vi "Start Live Mode.vi"(8 "error in (no error)":errorcluster, 10 "Camera Settings":T1={"Exposure Time (ms)"=100.0, "Binning"=enum."2x2", "Scan Mode"=0, "Frames to Acquire"=1000.0, "Pixel Correction"=FALSE, "Frames to Skip"=0, "File Path"=path "", "Duty cycle"=0.0, "ALEX"=FALSE, "Shutter Enable"=[], "fluidics trigger frame"=0, "Bit Depth"=0, "Image Width (px)"=0, "Image Height (px)"=0, "Horizontal Offset (px)"=0, "Vertical Offset (px)"=0} {"fluidics trigger frame" max=60000 step=1; "Exposure Time (ms)" min=1.0 max=10000.0 step=1.0}, 11 "Photometrics Camera in":refnum<class "Photometrics Camera.lvclass">) -> (0 "error out":errorcluster, 3 "Photometrics Camera out":refnum<class "Photometrics Camera.lvclass">)   [LabVIEW 2022 SP3, in "Photometrics Camera.lvlib" / "Photometrics Camera.lvclass"]
uses:
  Photometrics Camera.lvclass
  Resources/Type Defs/Camera Settings.ctl
  C:/FlashGordon/Development/dll/PVCamNET.dll
  dll/PVCamNET.dll
  Camera/Camera.lvclass
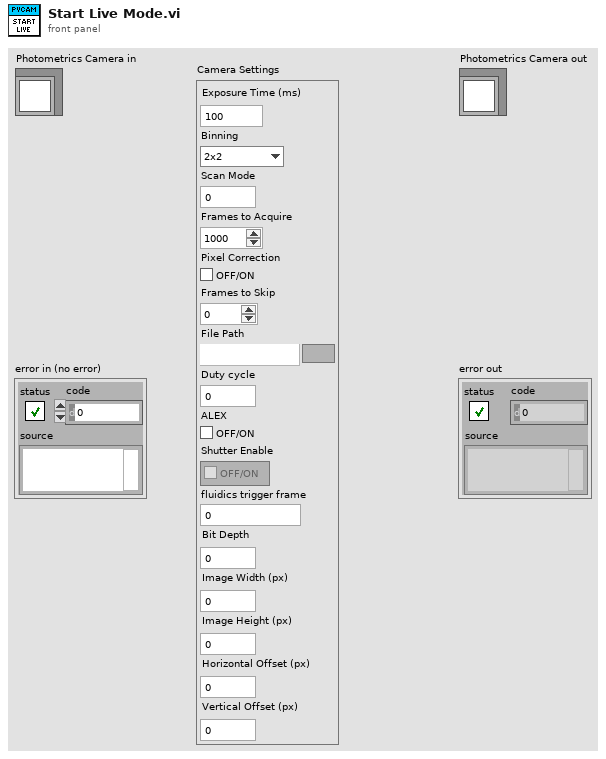
[diagram p1: front panel]
types:
  T1 = typedef "Camera Settings.ctl" = cluster{"Exposure Time (ms)":dbl, "Binning":enum16{"1x1", "2x2", "4x4"}, "Scan Mode":i32, "Frames to Acquire":dbl, "Pixel Correction":bool, "Frames to Skip":u32, "File Path":path, "Duty cycle":dbl, "ALEX":bool, "Shutter Enable":bool[], "fluidics trigger frame":u16, "Bit Depth":u16, "Image Width (px)":u16, "Image Height (px)":u16, "Horizontal Offset (px)":u16, "Vertical Offset (px)":u16}
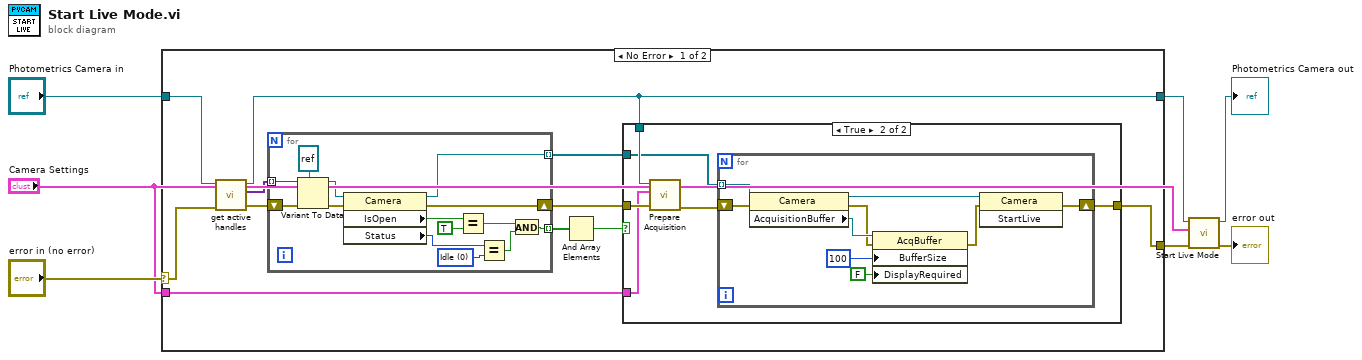
[diagram p0: block diagram]
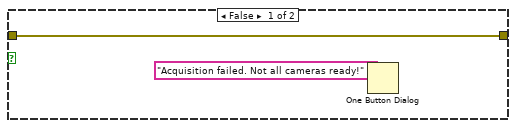
[diagram p2: hidden frame]
diagram:
  n1 = case shown="No Error" "error in (no error)" {
    selector: "error in (no error)" -> [w12 w51]
    tunnel: [w15 w51] -> w3
    tunnel: "Photometrics Camera in" -> [w11 w50]
    tunnel: [w10 w50] -> w2
    tunnel: "Camera Settings" -> [w14 _]
    frame No Error {
      n2 = call-dynamic "get active handles.vi"("error in (no error)"=w12, "Camera in"=w11) -> ("error out"=w13:errorcluster, "Handles"=w9:variant[], "Camera out"=w10:refnum<class "Photometrics Camera.lvclass">)  [unwired: 5 in, 2 out]
      n3 = for {
        tunnel: [w43] -> w17 mode=indexing
        tunnel: w9 -> [w40] mode=indexing
        shift-right: [w42] -> w18
        shift-left: w13 -> [w39]
        tunnel: [w41] -> w8 mode=indexing
        w48 = 0 items=["Idle", "Capturing"] ("Status")
        n4 = Variant To Data(error in=w39, type=refnum<k24> refnum ("reference out"), Variant=w40) -> (data=w37:refnum<k24>, error out=w38:errorcluster)
        n5 = property class="Camera"(reference=w37, error in=w38) -> (reference out=w41:refnum<k24>, error out=w42:errorcluster, "IsOpen"=w47:bool, "Status"=w49:i32)
        n6 = Equal?(x=w47, y=TRUE) -> (x = y?=w45:bool)
        n7 = Equal?(x=w49, y=w48) -> (x = y?=w44:bool)
        n8 = And(x=w45, y=w44) -> (x .and. y?=w43:bool)
      }
      n9 = And Array Elements(Boolean array=w17) -> (logical AND=w16:bool)
      n10 = case shown="True" w16 {
        tunnel: [w20 w26] -> w15
        tunnel: w18 -> [w20 w25]
        tunnel: w10 -> [_ w23]
        tunnel: w14 -> [_ w22]
        tunnel: w8 -> [_ w21]
        frame False {
          n11 = One Button Dialog(message="Acquisition failed. Not all cameras ready!") -> ()  [unwired: 1 in, 1 out]
        }
        frame True {
          n12 = call-dynamic "Prepare Acquisition.vi"("error in (no error)"=w25, "Camera Settings"=w22, "Photometrics Camera in"=w23) -> ("error out"=w24:errorcluster)  [unwired: 7 in, 1 out]
          n13 = for {
            tunnel: w21 -> [w34] mode=indexing
            shift-right: [w35] -> w26
            shift-left: w24 -> [w33]
            n14 = property class="Camera"(reference=w34, error in=w33) -> (reference out=w32:refnum<k24>, error out=w29:errorcluster, "AcquisitionBuffer"=w31:refnum<k24>)
            n15 = property class="AcqBuffer"(reference=w31, error in=w29, "BufferSize"=u32 100, "DisplayRequired"=FALSE ("UseScaling")) -> (error out=w27:errorcluster)  [unwired: 1 out]
            n16 = invoke class="Camera" method="StartLive"(reference=w32, error in=w27) -> (error out=w35:errorcluster)  [unwired: 1 in, 2 out]
          }
        }
      }
    }
    frame Error {
    }
  }
  n17 = call-parent "Start Live Mode.vi"("error in (no error)"=w3, "Camera Settings"="Camera Settings", "Camera in"=w2) -> ("error out"=→"error out":errorcluster, "Camera out"=→"Photometrics Camera out":refnum<class "Photometrics Camera.lvclass">)  [unwired: 7 in]
